vi "ToFieldCentric.vi"(10 "IMU Value (offset)":dbl, 11 "Rotation (degrees)":dbl[](array[numeric])) -> (3 "Heading":dbl)   [LabVIEW 2020]
uses:
  <vilib>/Analysis/coordinate.llb/Angle Units.ctl
  <vilib>/Analysis/coordinate.llb/Angle Range (Degree).ctl
  <vilib>/Analysis/coordinate.llb/Wrap Angle (scalar).vi
  <vilib>/Analysis/NI_AAL_Angle.lvlib
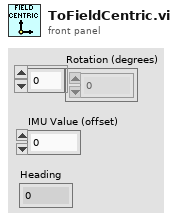
[diagram p1: front panel]
types:
  T1 = typedef "NI_AAL_Angle.lvlib/Angle Range (Degree).ctl" = u16
  T2 = typedef "NI_AAL_Angle.lvlib/Angle Units.ctl" = i32
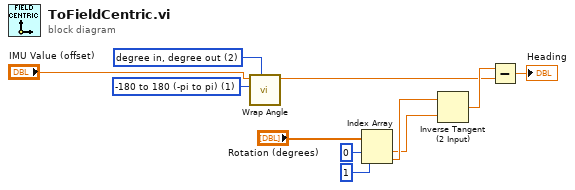
[diagram p0: block diagram]
diagram:
  w10 = T1 1 items=["none", "-180 to 180 (-pi to pi)", "0 to 360 (0 to 2pi)"] ("angle range")
  w11 = T2 2 items=["radian in, radian out", "radian in, degree out", "degree in, degree out", "degree in, radian out"] ("angle units")
  n1 = call-poly <vilib>:"Wrap Angle.vi"("angle units"=w11, "angle range"=w10, "angle in"="IMU Value (offset)") -> ("angle out"=w2:dbl)  [unwired: 7 in, 1 out]
  n2 = Index Array(array="Rotation (degrees)", index #1=0 ("index"), index #2=1 ("index")) -> (element #1=w4:dbl, element #2=w5:dbl)
  n3 = Inverse Tangent (2 Input)(1:w4, 2:w5) -> (0:w3:dbl)
  n4 = Subtract(x=w3, y=w2) -> (x-y=→"Heading":dbl)
